vi "Do Request.vi"(7 "Processing In":refnum<class "Processing.lvclass">, 11 "User API in":refnum<class "User API.lvclass">) -> (0 "error out":errorcluster, 5 "Processing":refnum<class "Processing.lvclass">)   [LabVIEW 2020, in "Summer of LabVIEW.lvlib" / "User API.lvclass"]
uses:
  User API.lvclass
  <vilib>/IlluminatedG/IG HTTP Server/HTTP Server/Processing/Processing.lvclass
  SOL User/SOL User.lvclass
  <vilib>/IlluminatedG/IG HTTP Server/HTTP Server/Security/Security.lvclass
  Data Types/User Info JSON.ctl
  <vilib>/IlluminatedG/IG HTTP Server/HTTP Server/Processing/Processing.lvclass/Processing.ctl
  700af4c1-b19f-4049-9cd2-76dfadd6391a.vi
  7b6a49e8-3e33-4c42-ba4f-db593ec10bd3.vi
  700af4c1-b19f-4049-9cd2-76dfadd6391a.vi/5a4e7add-6e55-453e-b5d5-028ac39578e6.vi
  7b6a49e8-3e33-4c42-ba4f-db593ec10bd3.vi/5a4e7add-6e55-453e-b5d5-028ac39578e6.vi
  700af4c1-b19f-4049-9cd2-76dfadd6391a.vi/5a4e7add-6e55-453e-b5d5-028ac39578e6.vi/9528e9df-aefc-4ce0-9221-106a337fd3b6.vi
  7b6a49e8-3e33-4c42-ba4f-db593ec10bd3.vi/5a4e7add-6e55-453e-b5d5-028ac39578e6.vi/9528e9df-aefc-4ce0-9221-106a337fd3b6.vi
  <vilib>/IlluminatedG/IG HTTP Server/HTTP Server/Processing/Get Values.vi
  <vilib>/IlluminatedG/IG HTTP Server/HTTP Server/Values/Get Arg Map.vi
  <vilib>/Utility/error.llb/Error Cluster From Error Code.vi
  User API.lvclass/User API.ctl
  Summer of LabVIEW.lvlib
  <vilib>/IlluminatedG/IG HTTP Utils/HTTP Utils/Response/Response.lvclass
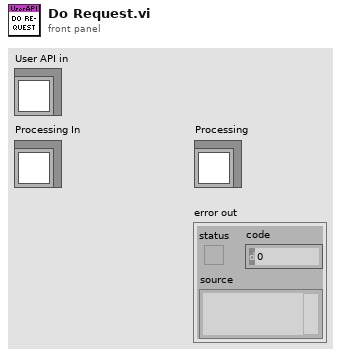
[diagram p1: front panel]
types:
  T1 = typedef "Summer of LabVIEW.lvlib/User Info JSON.ctl" = cluster{"email":string, "first_name":string, "last_name":string, "department":string, "admin":bool}
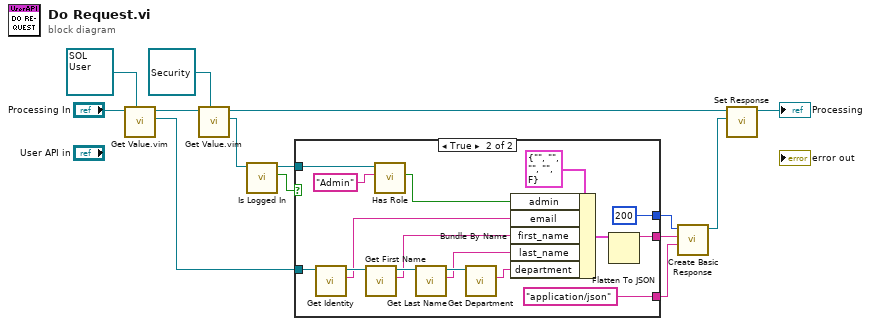
[diagram p0: block diagram]
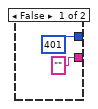
[diagram p2: hidden frame]
diagram:
  n1 = call "Get Value.vim"("Type / Server / Service (String)"=refnum<class "SOL User.lvclass"> refnum ("SOL:SOL User.lvclass"), "Processing in"="Processing In") -> ("Value"=w12:refnum<class "SOL User.lvclass">, "Processing out"=w9:refnum<class "Processing.lvclass">)  [unwired: 7 in, 1 out]
  n2 = call "Get Value.vim"("Type / Server / Service (String)"=refnum<class "Security.lvclass"> refnum ("HTTP Server.lvlib:Security.lvclass"), "Processing in"=w9) -> ("Value"=w7:refnum<class "Security.lvclass">, "Processing out"=w6:refnum<class "Processing.lvclass">)  [unwired: 7 in, 1 out]
  n3 = call <vilib>:"Is Logged In.vi"("Security in"=w7) -> ("Logged In"=w3:bool, "Security out"=w1:refnum<class "Security.lvclass">)  [unwired: 8 in, 1 out]
  n4 = case shown="True" w3 {
    tunnel: w12 -> [_ w32]
    tunnel: ["" ("JSON string") w31] -> w11
    tunnel: [u16 401 ("Status Code") u16 200 ("Status Code")] -> w10
    tunnel: [_ "application/json"] -> w2
    tunnel: w1 -> [_ w19]
    frame False {
    }
    frame True {
      n5 = call-dynamic "Get Identity.vi"("SOL User in"=w32) -> ("Identity"=w22:string, "SOL User out"=w29:refnum<class "SOL User.lvclass">)  [unwired: 8 in, 1 out]
      n6 = call "Get First Name.vi"("SOL User in"=w29) -> ("First Name"=w23:string, "SOL User out"=w28:refnum<class "SOL User.lvclass">)  [unwired: 8 in, 1 out]
      n7 = call <vilib>:"Has Role.vi"("Role"="Admin", "Security in"=w19) -> ("Has Role?"=w17:bool)  [unwired: 7 in, 2 out]
      n8 = call "Get Last Name.vi"("SOL User in"=w28) -> ("Last Name"=w24:string, "SOL User out"=w27:refnum<class "SOL User.lvclass">)  [unwired: 8 in, 1 out]
      n9 = call "Get Department.vi"("SOL User in"=w27) -> ("Department"=w25:string)  [unwired: 8 in, 2 out]
      n10 = Bundle By Name(cluster=T1 {"email"="", "first_name"="", "last_name"="", "department"="", "admin"=FALSE} ("User Info JSON"), "admin"=w17, "email"=w22, "first_name"=w23, "last_name"=w24, "department"=w25) -> (w21:T1)
      n11 = Flatten To JSON(anything=w21) -> (JSON string=w31:string)  [unwired: 2 in, 1 out]
    }
  }
  n12 = call <vilib>:"Create Basic Response.vi"("Content-Type (text/plain)"=w2, "Payload"=w11, "Status Code"=w10) -> ("Response out"=w4:refnum<class "Response.lvclass">)  [unwired: 7 in, 1 out]
  n13 = call <vilib>:"Set Response.vi"("Response"=w4, "Processing in"=w6) -> ("Processing out"=→"Processing":refnum<class "Processing.lvclass">)  [unwired: 9 in]
